vi "To Host FIFOs.vi"(0 "data":cluster{"Element":i16[]}[](array[cluster])=[{"Element"=[]}, {"Element"=[]}, {"Element"=[]}, {"Element"=[]}], 5 "data valid":bool[](array[boolean])=[FALSE, FALSE, FALSE, FALSE]) -> (13 "all ready for input":bool, 14 "each ready for input":bool[](array[boolean]))   [LabVIEW 2018, in "GettingStarted_5785_FPGA.lvlib"]
uses:
  GettingStarted_5785_FPGA.lvlib
  <vilib>/rvi/interface/RandomDataEmulation/nirviRandomDataMultiElementFPGAFIFO.vi
  <instcachedir>/0/nirviRandomDataMultiElementFPGAFIFO_6740B454F3C245F78F76ED91F73FD8DB.lvgen/nirviRandomDataMultiElementFPGAFIFO_6740B454F3C245F78F76ED91F73FD8DB_002.vi
  <vilib>/rvi/interface/RandomDataEmulation/niFpgaRandomDataHandleErrors.vi
  <vilib>/rvi/DataTransferAndStorage/Container/XNode/niFpgaContainer.xnode
  <vilib>/rvi/interface/RandomDataEmulation/nirviRandomDataFpgaMultiElementTemplate.vi
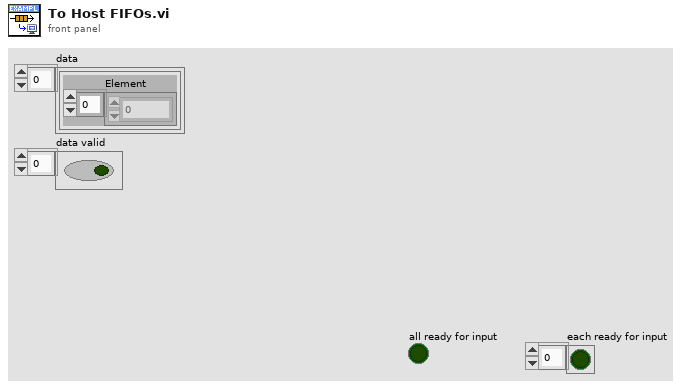
[diagram p1: front panel]
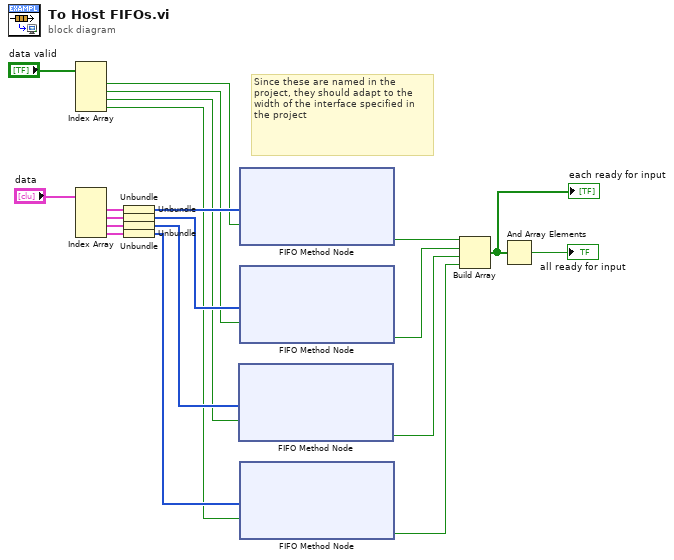
[diagram p0: block diagram]
diagram:
  # "Since these are named in the project, they should adapt to the width of the interface specified in the project"
  n1 = Index Array(array="data valid") -> (element #1=w4:bool, element #2=w3:bool, element #3=w2:bool, element #4=w1:bool)  [unwired: 4 in]
  n2 = Index Array(array="data") -> (element #1=w13:cluster{"Element":i16[]}, element #2=w11:cluster{"Element":i16[]}, element #3=w8:cluster{"Element":i16[]}, element #4=w9:cluster{"Element":i16[]})  [unwired: 4 in]
  n3 = Unbundle(w13) -> ("Element"=w12:i16[])
  n4 = Unbundle(w11) -> ("Element"=w10:i16[])
  n5 = Unbundle(w8) -> ("Element"=w7:i16[])
  n6 = Unbundle(w9) -> ("Element"=w6:i16[])
  n7 = xnode ("FIFO Method Node")("Element"=w7, "Input Valid"=w2) -> ("Ready for Input"=w18:bool)  [unwired: 1 in, 1 out]
  n8 = xnode ("FIFO Method Node")("Element"=w12, "Input Valid"=w4) -> ("Ready for Input"=w20:bool)  [unwired: 1 in, 1 out]
  n9 = xnode ("FIFO Method Node")("Element"=w10, "Input Valid"=w3) -> ("Ready for Input"=w19:bool)  [unwired: 1 in, 1 out]
  n10 = xnode ("FIFO Method Node")("Element"=w6, "Input Valid"=w1) -> ("Ready for Input"=w17:bool)  [unwired: 1 in, 1 out]
  n11 = Build Array(w20, w19, w18, w17) -> (w16:bool[])
  "each ready for input" <- w16
  n12 = And Array Elements(Boolean array=w16) -> (logical AND=→"all ready for input":bool)
